vi "Bits limits.vi"() -> ()   [LabVIEW 2015]
panel:
  in  "X 4":i32 format="%d (0x%x) (b%032b)"
  in  "X 3":i32 format="%d (0x%x) (b%b)"
  out "Y (U)":u8 format="%d (0x%x) (b%b)"
  out "-2^(n-1)":i8 format="%d (0x%x) (b%b)"
  in  "N":i32 format="%d (0x%x) (b%b)"
  out "2^(n-1)-1":i8 format="%d (0x%x) (b%b)"
  out "Y (I)":i8 format="%d (0x%x) (b%b)"
  in  "X 2":i8 format="%d (0x%x) (b%b)"
  in  "X":i8 format="%d (0x%x) (b%b)"
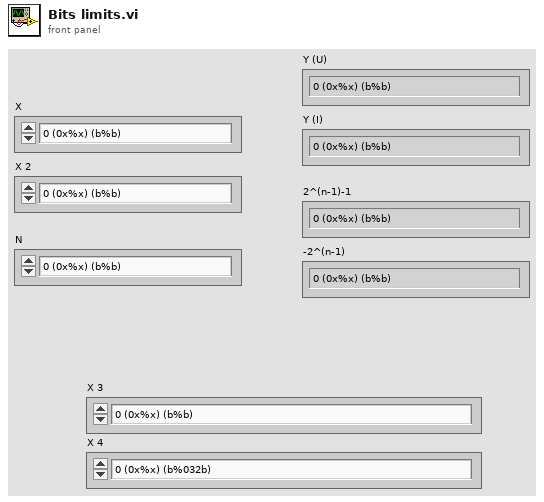
[diagram p1: front panel]
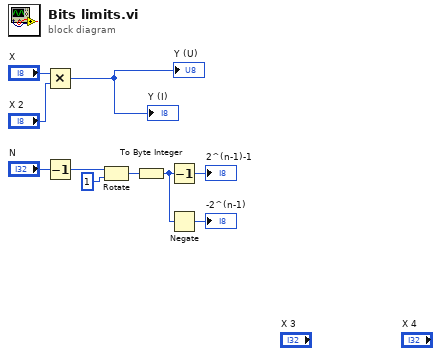
[diagram p0: block diagram]
diagram:
  n1 = Multiply(x="X", y="X 2") -> (x*y=→"Y (I)" →"Y (U)":i8)
  n2 = Decrement(x="N") -> (x-1=w2:i32)
  n3 = Rotate(1:i8 1 ("y"), 2:w2) -> (0:w6:i8)
  n4 = To Byte Integer(number=w6) -> (8bit integer=w4:i8)
  n5 = Decrement(x=w4) -> (x-1=→"2^(n-1)-1":i8)
  n6 = Negate(x=w4) -> (-x=→"-2^(n-1)":i8)
